vi "disableHardware.vi"(0 "error in (no error)":errorcluster, 1 "Tension Sensors":refnum<k21>, 2 "Voltage Out":refnum<k21>, 3 "Encoders Task":refnum<k21>[](array[refnum])) -> ()   [LabVIEW 2013]
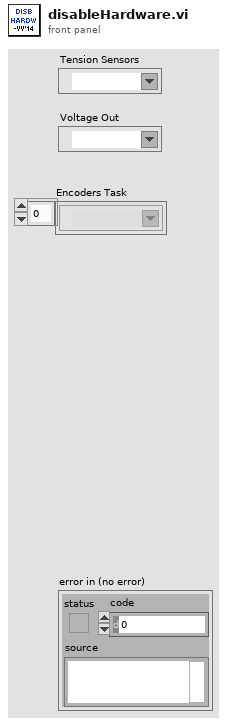
[diagram p1: front panel]
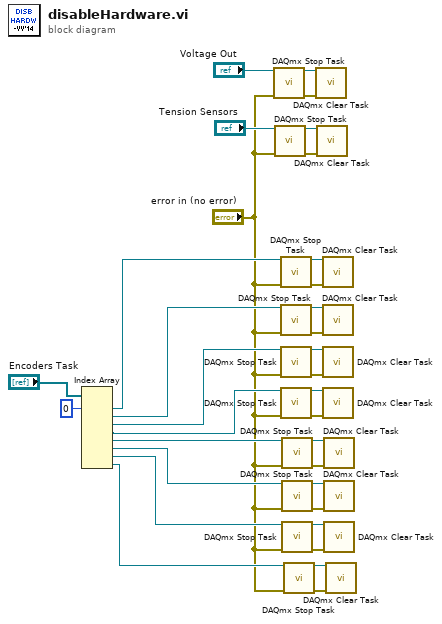
[diagram p0: block diagram]
diagram:
  n1 = Index Array(array="Encoders Task", index #1=0 ("index")) -> (element #1=w7:refnum<k21>, element #2=w8:refnum<k21>, element #3=w9:refnum<k21>, element #4=w10:refnum<k21>, element #5=w11:refnum<k21>, element #6=w12:refnum<k21>, element #7=w13:refnum<k21>, element #8=w2:refnum<k21>)  [unwired: 7 in]
  n2 = call <vilib>:"DAQmx Stop Task.vi"("task/channels in"="Voltage Out", "error in"="error in (no error)") -> ("task out"=w17:refnum<k21>, "error out"=w16:errorcluster)  [unwired: 12 in]
  n3 = call <vilib>:"DAQmx Stop Task.vi"("task/channels in"="Tension Sensors", "error in"="error in (no error)") -> ("task out"=w14:refnum<k21>, "error out"=w15:errorcluster)  [unwired: 12 in]
  n4 = call <vilib>:"DAQmx Stop Task.vi"("task/channels in"=w7, "error in"="error in (no error)") -> ("task out"=w21:refnum<k21>, "error out"=w20:errorcluster)  [unwired: 12 in]
  n5 = call <vilib>:"DAQmx Stop Task.vi"("task/channels in"=w8, "error in"="error in (no error)") -> ("task out"=w18:refnum<k21>, "error out"=w19:errorcluster)  [unwired: 12 in]
  n6 = call <vilib>:"DAQmx Stop Task.vi"("task/channels in"=w9, "error in"="error in (no error)") -> ("task out"=w29:refnum<k21>, "error out"=w28:errorcluster)  [unwired: 12 in]
  n7 = call <vilib>:"DAQmx Stop Task.vi"("task/channels in"=w10, "error in"="error in (no error)") -> ("task out"=w26:refnum<k21>, "error out"=w27:errorcluster)  [unwired: 12 in]
  n8 = call <vilib>:"DAQmx Stop Task.vi"("task/channels in"=w11, "error in"="error in (no error)") -> ("task out"=w22:refnum<k21>, "error out"=w23:errorcluster)  [unwired: 12 in]
  n9 = call <vilib>:"DAQmx Stop Task.vi"("task/channels in"=w12, "error in"="error in (no error)") -> ("task out"=w25:refnum<k21>, "error out"=w24:errorcluster)  [unwired: 12 in]
  n10 = call <vilib>:"DAQmx Stop Task.vi"("task/channels in"=w13, "error in"="error in (no error)") -> ("task out"=w30:refnum<k21>, "error out"=w31:errorcluster)  [unwired: 12 in]
  n11 = call <vilib>:"DAQmx Stop Task.vi"("task/channels in"=w2, "error in"="error in (no error)") -> ("task out"=w4:refnum<k21>, "error out"=w3:errorcluster)  [unwired: 12 in]
  n12 = call <vilib>:"DAQmx Clear Task.vi"("task in"=w17, "error in"=w16) -> ()  [unwired: 13 in, 1 out]
  n13 = call <vilib>:"DAQmx Clear Task.vi"("task in"=w14, "error in"=w15) -> ()  [unwired: 13 in, 1 out]
  n14 = call <vilib>:"DAQmx Clear Task.vi"("task in"=w21, "error in"=w20) -> ()  [unwired: 13 in, 1 out]
  n15 = call <vilib>:"DAQmx Clear Task.vi"("task in"=w18, "error in"=w19) -> ()  [unwired: 13 in, 1 out]
  n16 = call <vilib>:"DAQmx Clear Task.vi"("task in"=w29, "error in"=w28) -> ()  [unwired: 13 in, 1 out]
  n17 = call <vilib>:"DAQmx Clear Task.vi"("task in"=w26, "error in"=w27) -> ()  [unwired: 13 in, 1 out]
  n18 = call <vilib>:"DAQmx Clear Task.vi"("task in"=w22, "error in"=w23) -> ()  [unwired: 13 in, 1 out]
  n19 = call <vilib>:"DAQmx Clear Task.vi"("task in"=w25, "error in"=w24) -> ()  [unwired: 13 in, 1 out]
  n20 = call <vilib>:"DAQmx Clear Task.vi"("task in"=w30, "error in"=w31) -> ()  [unwired: 13 in, 1 out]
  n21 = call <vilib>:"DAQmx Clear Task.vi"("task in"=w4, "error in"=w3) -> ()  [unwired: 13 in, 1 out]
